vi "AGdll.vi"(8 "error in (no error)":errorcluster, 11 "Input Cluster":cluster{"t":dbl, "d":dbl, "z":dbl[]}={"t"=0.0, "d"=0.0, "z"=[0.0, 0.0, 0.0, 0.0, 0.0, 0.0, 0.0, 0.0, 0.0, 0.0, 0.0, 0.0, 0.0, 0.0, 0.0, 0.0, 0.0, 0.0, 0.0, 0.0]}) -> (0 "error out":errorcluster, 3 "Output Cluster":cluster{"a":dbl, "g":dbl})   [LabVIEW 2021]
doc: "subroutine AGdll(t, d, z, a, g)\nCompute Helmholtz and Gibbs energies as functions of temperature, density, and composition. These are not\nresidual values (those are calculated by GIBBS). See warning in suroutines THERM or ALLPROPS.\n\nINPUTS:\n t -- Temperature [K]\n d -- Molar density [mol/L]\n z -- Composition (array of mole fractions)\n\nOUTPUTS:\n a -- Helmholtz energy [J/mol]\n g -- Gibbs free energy [J/mol}"
uses:
  REFPROP.dll
panel:
  # "REFPROP-AGdll.vi"
  # "subroutine AGdll(t, d, z, a, g)"
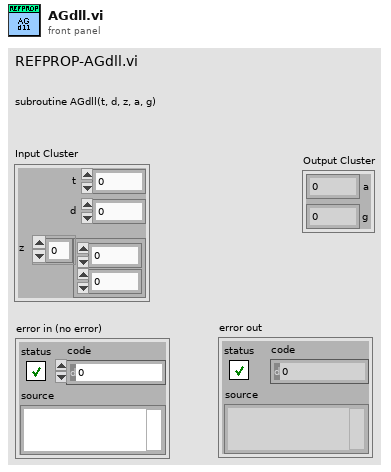
[diagram p1: front panel]
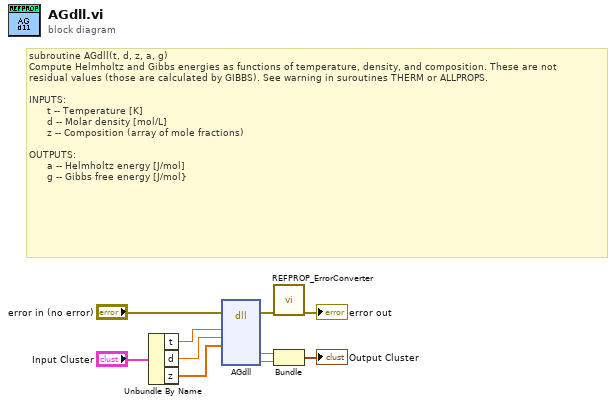
[diagram p0: block diagram]
diagram:
  # "subroutine AGdll(t, d, z, a, g)\nCompute Helmholtz and Gibbs energies as functions of temperature, density, and composition. These are not\nresidual values (those are calculated by GIBBS). See warning in suroutines THERM or ALLPROPS.\n\nINPUTS:\n      t -- Temperature [K]\n      d -- Molar density [mol/L]\n      z -- Composition (array of mole fractions)\n\nOUTPUTS:\n      a -- Helmholtz energy [J/mol]\n      g -- Gibbs free energy [J/mol}"
  n1 = Unbundle By Name("Input Cluster") -> ("t"=w6:dbl, "d"=w5:dbl, "z"=w4:dbl[])
  n2 = dll-call lib="C:/Users/lauria/OneDrive - National Institute of Standards and Technology (NIST)/LabVIEW Projects/7 REFPROP/REFPROP-wrappers-master/REFPROP-wrappers-master/wrappers/Labview/REFPROP/REFPROP.*" fn="AGdll"(error in="error in (no error)", "t"=w6, "d"=w5, "z"=w4) -> (error out=w10:errorcluster, "a"=w3:dbl, "g"=w2:dbl)  [unwired: 8 in, 1 out]
  n3 = call "REFPROP_ErrorConverter.vi"("error in (no error)"=w10) -> ("error out"=→"error out":errorcluster)  [unwired: 10 in]
  n4 = Bundle("a"=w3, "g"=w2) -> (→"Output Cluster":cluster{"a":dbl, "g":dbl})  [unwired: 1 in]
